vi "Change Window.vi"(8 "error in":errorcluster, 11 "WindowName":string) -> (0 "error out":errorcluster)   [LabVIEW 2020]
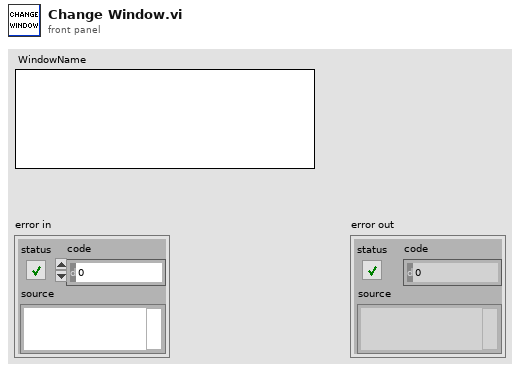
[diagram p1: front panel]
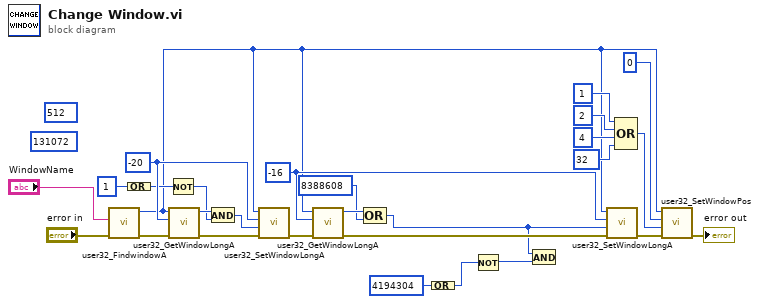
[diagram p0: block diagram]
diagram:
  (unwired) 131072 ("y")
  (unwired) 512 ("y")
  w10 = -16 ("nIndex")
  w25 = -20 ("nIndex")
  n1 = call "user32_FindwindowA.vi"("error in (no error)"="error in", "lpWindowName"="WindowName") -> ("error out"=w28:errorcluster, "Return"=w9:u32)  [unwired: 8 in]
  n2 = Compound Arithmetic op=OR(1 ("y")) -> (w21:i32)
  n3 = Not(x=w21) -> (.not. x?=w5:i32)
  n4 = call "user32_GetWindowLongA.vi"("error in (no error)"=w28, "nIndex"=w25, "hWnd"=w9) -> ("error out"=w27:errorcluster, "return"=w26:i32)  [unwired: 7 in]
  n5 = And(x=w26, y=w5) -> (x .and. y?=w7:i32)
  n6 = call "user32_SetWindowLongA.vi"("error in (no error)"=w27, "dwNewLong"=w7, "nIndex"=w25, "hWnd"=w9) -> ("error out"=w12:errorcluster)  [unwired: 6 in, 1 out]
  n7 = call "user32_GetWindowLongA.vi"("error in (no error)"=w12, "nIndex"=w10, "hWnd"=w9) -> ("error out"=w11:errorcluster, "return"=w8:i32)  [unwired: 7 in]
  n8 = Compound Arithmetic op=OR(w8, 8388608 ("value")) -> (w1:i32)
  n9 = Compound Arithmetic op=OR(4194304 ("y")) -> (w3:i32)
  n10 = Not(x=w3) -> (.not. x?=w2:i32)
  n11 = And(x=w1, y=w2) -> ()  [unwired: 1 out]
  n12 = call "user32_SetWindowLongA.vi"("error in (no error)"=w11, "dwNewLong"=w1, "nIndex"=w10, "hWnd"=w9) -> ("error out"=w13:errorcluster)  [unwired: 6 in, 1 out]
  n13 = Compound Arithmetic op=OR(1 ("y"), 2 ("y"), 4 ("y"), 32 ("y")) -> (w16:i32)
  n14 = call "user32_SetWindowPos.vi"("error in (no error)"=w13, "uFlags"=w16, "hWndInsertAfter"=i64 0, "hWnd"=w9) -> ("error out"=→"error out":errorcluster)  [unwired: 6 in, 1 out]
